vi "Create Shipping List.vi"(6 "Weight [kg]":dbl, 7 "Delivery Type":T2, 8 "error in (no error)":errorcluster, 9 "Recipient Data":T1, 10 "Sender Data":T1, 11 "Factory in":refnum<class "Factory.lvclass">) -> (0 "error out":errorcluster, 3 "Factory out":refnum<class "Factory.lvclass">)   [LabVIEW 2019, in "Factory.lvclass"]
uses:
  Factory.lvclass
  Controls/#enum_DeliveryType.ctl
  Controls/#cluster_PersonalData.ctl
  Delivery/Post/Post.lvclass
  C:/Users/Extensa/Desktop/Fabryka/Fabryka Rozwiazanie/Delivery/Delivery/Delivery.lvclass
  Factory.lvclass/Factory.ctl
  Delivery/Post/Post.lvclass/Post.ctl
  Delivery/Courier/Courier.lvclass
  Delivery/Pigeon/Pigeon.lvclass
  Delivery/Pigeon/Pigeon.lvclass/Pigeon.ctl
  Delivery/Delivery/Delivery.lvclass
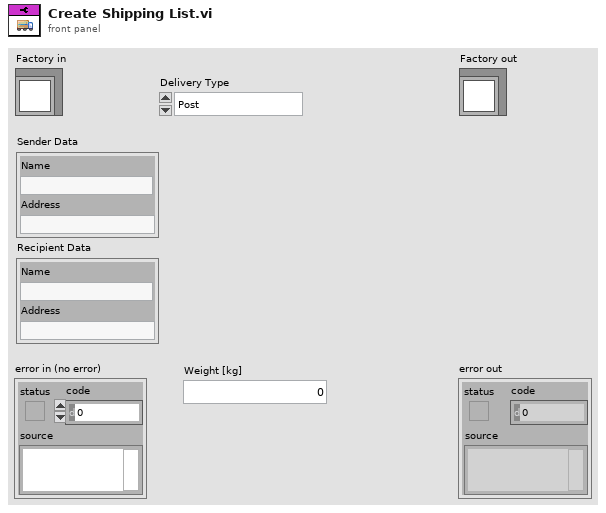
[diagram p1: front panel]
types:
  T1 = typedef "#cluster_PersonalData.ctl" = cluster{"Name":string, "Address":string}
  T2 = typedef "#enum_DeliveryType.ctl" = enum16{"Post", "Courier", "Pigeon"}
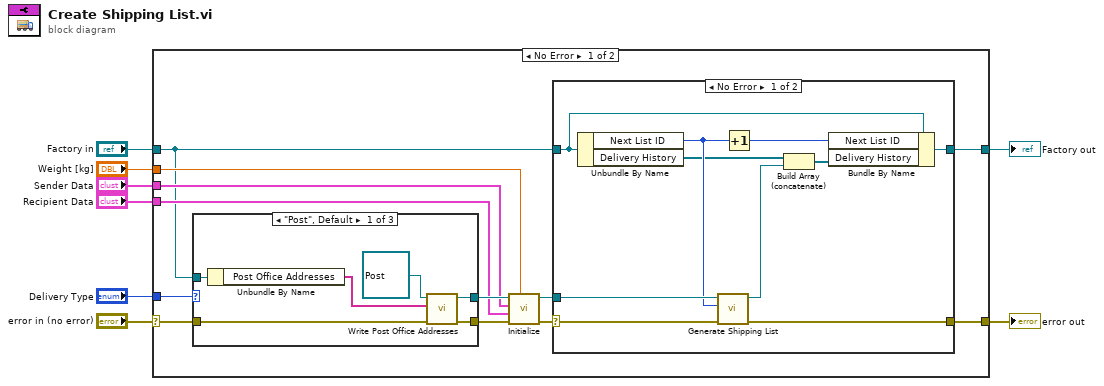
[diagram p0: block diagram]
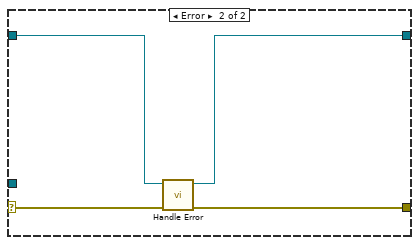
[diagram p2: hidden frame]
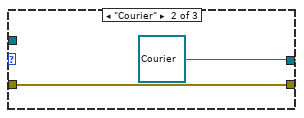
[diagram p3: hidden frame]
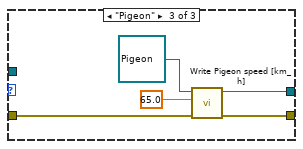
[diagram p4: hidden frame]
diagram:
  n1 = case shown="No Error" "error in (no error)" {
    selector: "error in (no error)" -> [w19 w49]
    tunnel: [w11 w49] -> w7
    tunnel: [w10 w48] -> w5
    tunnel: "Factory in" -> [w9 w48]
    tunnel: "Delivery Type" -> [w20 _]
    tunnel: "Weight [kg]" -> [w14 _]
    tunnel: "Sender Data" -> [w16 _]
    tunnel: "Recipient Data" -> [w15 _]
    frame No Error {
      n2 = case shown="\"Post\", Default" w20 {
        tunnel: w19 -> [w39 w42 w47]
        tunnel: [w38 w42 w44] -> w18
        tunnel: [w37 refnum<class "Courier.lvclass"> refnum ("Courier.lvclass") w43] -> w17
        tunnel: w9 -> [w40 _ _]
        frame "Post", Default {
          n3 = Unbundle By Name(w40) -> ("Post Office Addresses"=w35:string[])
          n4 = call "Write Post Office Addresses.vi"("error in (no error)"=w39, "Post Office Addresses"=w35, "Post in"=refnum<class "Post.lvclass"> refnum ("Post.lvclass")) -> ("error out"=w38:errorcluster, "Post out"=w37:refnum<class "Post.lvclass">)  [unwired: 7 in]
        }
        frame "Courier" {
        }
        frame "Pigeon" {
          n5 = call "Write Pigeon speed [km_h].vi"("error in (no error)"=w47, "Pigeon speed [km/h]"=65.0, "Pigeon in"=refnum<class "Pigeon.lvclass"> refnum ("Pigeon.lvclass")) -> ("error out"=w44:errorcluster, "Pigeon out"=w43:refnum<class "Pigeon.lvclass">)  [unwired: 7 in]
        }
      }
      n6 = call-dynamic "Initialize.vi"("Parcel Weight [kg]"=w14, "error in (no error)"=w18, "Recipient Data"=w15, "Sender Data"=w16, "Delivery in"=w17) -> ("error out"=w13:errorcluster, "Delivery out"=w12:refnum<class "Delivery.lvclass">)  [unwired: 5 in]
      n7 = case shown="No Error" w13 {
        selector: w13 -> [w30 w34]
        tunnel: w12 -> [w29 _]
        tunnel: w9 -> [w24 w33]
        tunnel: [w25 w32] -> w11
        tunnel: [w27 w31] -> w10
        frame No Error {
          n8 = Unbundle By Name(w24) -> ("Next List ID"=w26:i32, "Delivery History"=w23:refnum<class "Delivery.lvclass">[])
          n9 = call-dynamic "Generate Shipping List.vi"("error in (no error)"=w30, "Shipping ID"=w26, "Delivery in"=w29) -> ("error out"=w25:errorcluster, "Delivery out"=w22:refnum<class "Delivery.lvclass">)  [unwired: 7 in]
          n10 = Increment(x=w26) -> (x+1=w28:i32)
          n11 = Build Array (concatenate)(w23, w22) -> (w21:refnum<class "Delivery.lvclass">[])
          n12 = Bundle By Name(cluster=w24, "Next List ID"=w28, "Delivery History"=w21) -> (w27:refnum<class "Factory.lvclass">)
        }
        frame Error {
          n13 = call "Handle Error.vi"("error in (no error)"=w34, "Factory in"=w33) -> ("error out"=w32:errorcluster, "Factory out"=w31:refnum<class "Factory.lvclass">)  [unwired: 8 in]
        }
      }
    }
    frame Error {
    }
  }
  "error out" <- w7
  "Factory out" <- w5
